vi "MenuSelect.vi"(1 "Combo Bpx":refnum<vi>, 5 "error in":errorcluster, 9 "Data":string[](array[string]), 12 "OK":refnum<vi>, 13 "stop":refnum<vi>, 14 "Caption":string="Please Select Element") -> (6 "error out":errorcluster, 10 "Value":string)   [LabVIEW 2018, in "PNA-X.lvlib"]
uses:
  PNA-X.lvlib
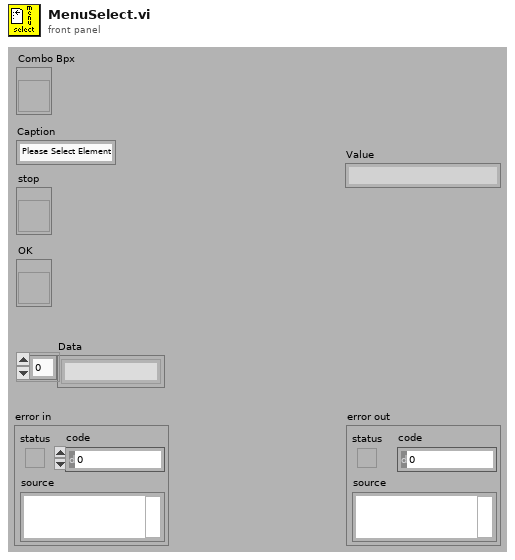
[diagram p1: front panel]
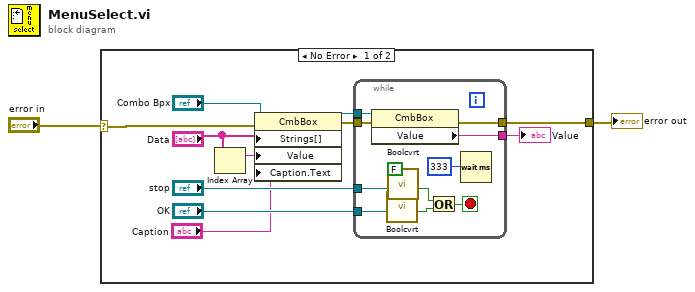
[diagram p0: block diagram]
diagram:
  n1 = case shown="No Error" "error in" {
    selector: "error in" -> [w3 w25]
    tunnel: [w11 w25] -> w2
    frame No Error {
      n2 = Index Array(array="Data") -> (element=w9:string)  [unwired: 1 in]
      n3 = property class="CmbBox"(reference="Combo Bpx", error in=w3, "Strings[]"="Data", "Value"=w9, "Caption.Text"="Caption") -> (reference out=w5:refnum<vi>, error out=w10:errorcluster)
      n4 = while {
        tunnel: [w24] -> w13
        tunnel: [w23] -> w11
        tunnel: "OK" -> [w19]
        tunnel: "stop" -> [w18]
        tunnel: w10 -> [w16]
        tunnel: w5 -> [w15]
        stop <- w20 stop-if-true
        n5 = property class="CmbBox"(reference=w15, error in=w16) -> (error out=w23:errorcluster, "Value"=w24:string)  [unwired: 1 out]
        n6 = call "Boolcvrt.vi"("Bool Refnum"=w19) -> ("T/F"=w21:bool)  [unwired: 9 in, 1 out]
        n7 = call "Boolcvrt.vi"("ORide"=FALSE, "Bool Refnum"=w18) -> ("T/F"=w22:bool)  [unwired: 8 in, 1 out]
        n8 = Or(x=w22, y=w21) -> (x .or. y?=w20:bool)
        n9 = Wait (ms)(milliseconds to wait=u32 333) -> ()  [unwired: 1 out]
      }
      "Value" <- w13
    }
    frame Error {
    }
  }
  "error out" <- w2
